vi "Cluster to Element Details.vi"(8 "error in":errorcluster, 11 "Cluster":variant) -> (0 "error out":errorcluster, 2 "More Cluster":variant[](array[variant]), 3 "gRPC Message Metadata":T1)   [LabVIEW 2019, in "gprc-lvsupport.lvlib"]
uses:
  gprc-lvsupport.lvlib
  typeDefs/Message Metadata.ctl
  typeDefs/Message Element Metadata.ctl
  typeDefs/Message Element Type.ctl
  <vilib>/Utility/Data Type/Type Definitions/Data Type.ctl
  <vilib>/Utility/Data Type/NI_Data Type.lvlib
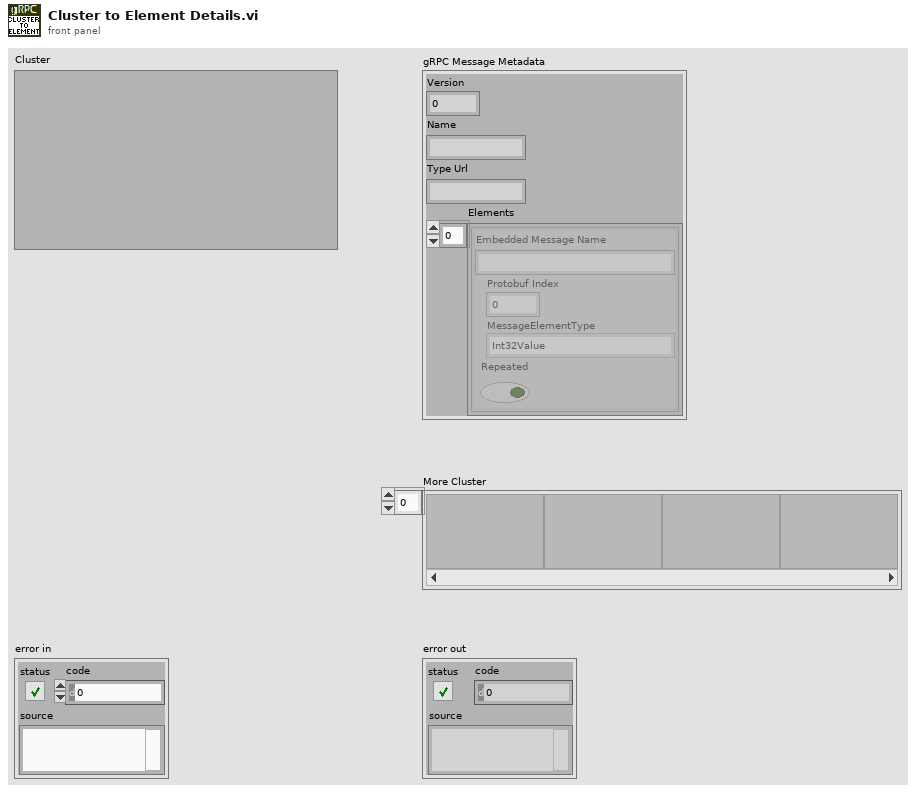
[diagram p1: front panel]
types:
  T1 = typedef "gprc-lvsupport.lvlib/Message Metadata.ctl" = cluster{"Version":i32, "Name":string, "Type Url":string, "Elements":T2[]}
  T2 = typedef "gprc-lvsupport.lvlib/Message Element Metadata.ctl" = cluster{"Embedded Message Name":string, "Protobuf Index":i32, "MessageElementType":T3, "Repeated":bool}
  T3 = typedef "gprc-lvsupport.lvlib/Message Element Type.ctl" = enum32{"Int32Value", "FloatValue", "DoubleValue", "BoolValue", "StringValue", "MessageValue", "Int64Value", "UInt32Value", "UInt64Value", "EnumValue", "Bytes", "Fixed64", "Fixed32", "SFixed64", "SFixed32", "SInt64", "SInt32"}
  T4 = typedef "NI_Data Type.lvlib/Data Type.ctl" = enum8{"Invalid Type", "Void", "I8", "I16", "I32", "I64", "U8", "U16", "U32", "U64", "Single Float", "Double Float", "Extended Float", "Single Complex", "Double Complex", "Extended Complex", "Enum U8", "Enum U16", "Enum U32", "Enum U64", "Single Float With Unit", "Double Float With Unit", "Extended Float With Unit", "Single Complex with Unit", "Double Complex with Unit", "Extended Complex with Unit", "Boolean", "String", "Path", "Picture", "Tag", "Array", "Cluster", "Variant", "LV Variant", "Waveform", "Timestamp", "Digital Waveform", "Digital Data", "ExpressData", "Refnum", "External Data", "VI", "Poly VI", "LabVIEW Class Instance", "Fixed Point", "Set Collection", "Map Collection"}
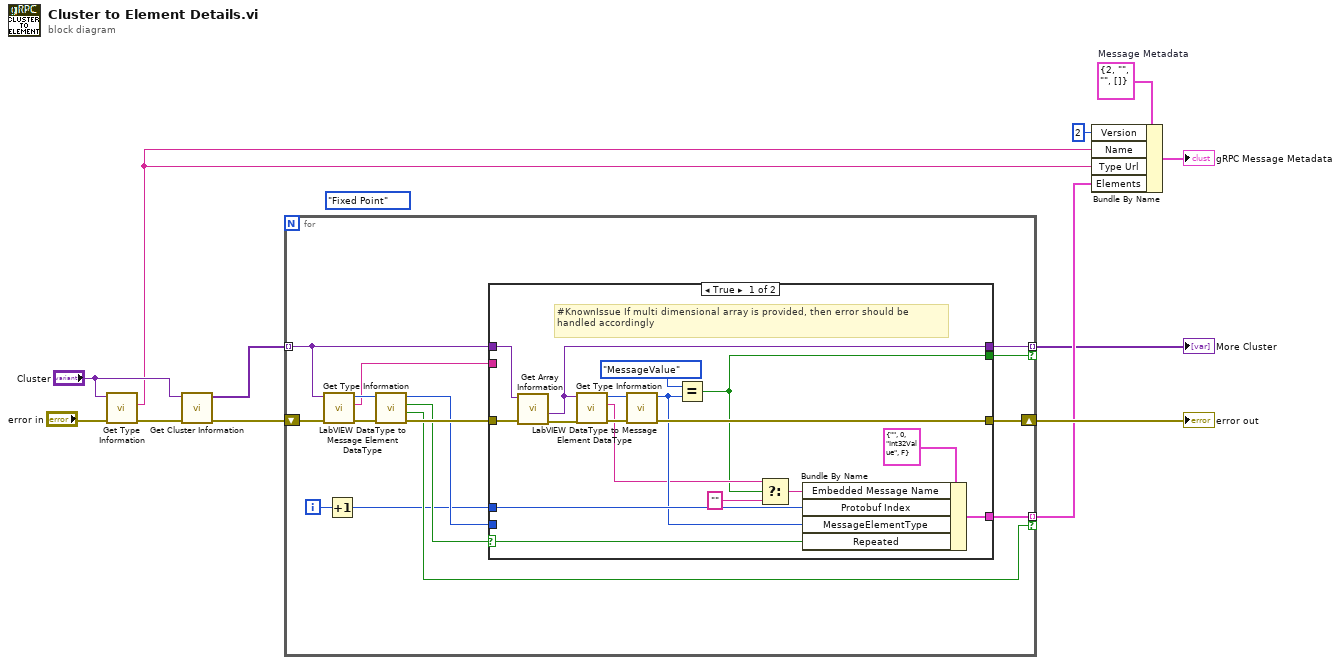
[diagram p0: block diagram]
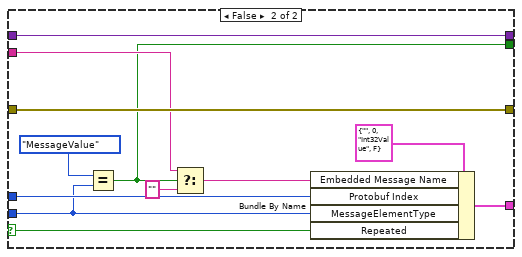
[diagram p2: hidden frame]
diagram:
  (unwired) Data_Type."Fixed Point" ("type")
  w8 = T1 {"Version"=2, "Name"="", "Type Url"="", "Elements"=[]}  # Message Metadata
  n1 = call <vilib>:"Get Type Information.vi"("error in (no error)"="error in", "variant"="Cluster") -> ("error out"=w12:errorcluster, "name"=w4:string)  [unwired: 5 in, 3 out]
  n2 = call <vilib>:"Get Cluster Information.vi"("error in (no error)"=w12, "variant"="Cluster") -> ("error out"=w11:errorcluster, "cluster elements"=w5:variant[])  [unwired: 8 in]
  n3 = for {
    tunnel: w5 -> [w17] mode=indexing
    tunnel: [w19] -> w3 mode=indexing if=w18
    shift-right: [w24] -> w10
    shift-left: w11 -> [w27]
    tunnel: [w14] -> w2 mode=indexing if=w13
    i -> [w23]
    n4 = call <vilib>:"Get Type Information.vi"("error in (no error)"=w27, "variant"=w17) -> ("error out"=w26:errorcluster, "name"=w15:string, "type"=w22:T4)  [unwired: 5 in, 2 out]
    n5 = Increment(x=w23) -> (x+1=w16:i32)
    n6 = call "LabVIEW DataType to Message Element DataType.vi"("error in"=w26, "type"=w22) -> ("error out"=w25:errorcluster, "Supported?"=w18:bool, "Array?"=w20:bool, "MessageElementType"=w21:T3)  [unwired: 6 in]
    n7 = case shown="True" w20 {
      selector: w20 -> [w38 w53]
      tunnel: w16 -> [w40 w55]
      tunnel: w21 -> [_ w51]
      tunnel: [w37 w52] -> w19
      tunnel: w25 -> [w44 w56]
      tunnel: w17 -> [w36 w46]
      tunnel: [w41 w56] -> w24
      tunnel: w15 -> [_ w49]
      tunnel: [w28 w46] -> w14
      tunnel: [w29 w45] -> w13
      frame True {
        # "#KnownIssue If multi dimensional array is provided, then error should be handled accordingly"
        n8 = call <vilib>:"Get Array Information.vi"("error in (no error)"=w44, "variant"=w36) -> ("error out"=w43:errorcluster, "array element data type"=w28:variant)  [unwired: 6 in, 2 out]
        n9 = call <vilib>:"Get Type Information.vi"("error in (no error)"=w43, "variant"=w28) -> ("error out"=w42:errorcluster, "name"=w31:string, "type"=w35:T4)  [unwired: 5 in, 2 out]
        n10 = call "LabVIEW DataType to Message Element DataType.vi"("error in"=w42, "type"=w35) -> ("error out"=w41:errorcluster, "MessageElementType"=w32:T3)  [unwired: 6 in, 2 out]
        n11 = Equal?(x=Message_Element_Type."MessageValue", y=w32) -> (x = y?=w29:bool)
        n12 = Select(t=w31, s=w29, f="") -> (s? t:f=w30:string)
        n13 = Bundle By Name(cluster=T2 {"Embedded Message Name"="", "Protobuf Index"=0, "MessageElementType"=enum."Int32Value", "Repeated"=FALSE} ("MessageElementMetadata"), "Embedded Message Name"=w30, "Protobuf Index"=w40, "MessageElementType"=w32, "Repeated"=w38) -> (w37:T2)
      }
      frame False {
        n14 = Equal?(x=Message_Element_Type."MessageValue", y=w51) -> (x = y?=w45:bool)
        n15 = Select(t=w49, s=w45, f="") -> (s? t:f=w48:string)
        n16 = Bundle By Name(cluster=T2 {"Embedded Message Name"="", "Protobuf Index"=0, "MessageElementType"=enum."Int32Value", "Repeated"=FALSE} ("MessageElementMetadata"), "Embedded Message Name"=w48, "Protobuf Index"=w55, "MessageElementType"=w51, "Repeated"=w53) -> (w52:T2)
      }
    }
  }
  "More Cluster" <- w2
  "error out" <- w10
  n17 = Bundle By Name(cluster=w8, "Version"=2, "Name"=w4, "Type Url"=w4, "Elements"=w3) -> (→"gRPC Message Metadata":T1)
